vi "Config Read Part Type.vi"(8 "Error In":errorcluster) -> (0 "Error Out":errorcluster, 1 "Part Infos":T1[](array[typedef]), 3 "Part Types":string[](array[string]))   [LabVIEW 2018]
uses:
  type defs/EOL Part Setup.ctl
  02.Type Def's/All Communication Types.ctl
  type defs/Communication with Motors.ctl
  type defs/RAP Signal Control.ctl
  type defs/EOL Motor Type.ctl
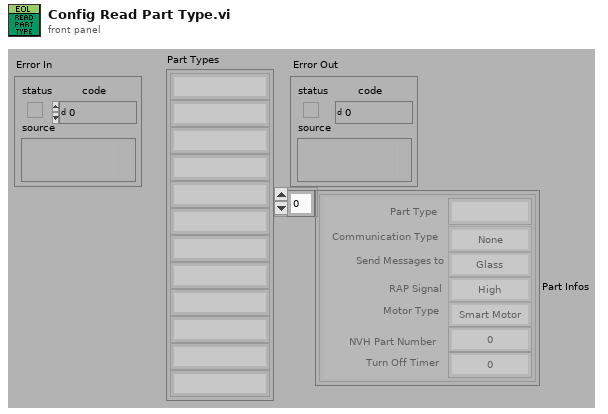
[diagram p1: front panel]
types:
  T1 = typedef "EOL Part Setup.ctl" = cluster{"Communication Type":T2, "Send Messages to":T3, "RAP Signal":T4, "Motor Type":T5, "NVH Part Number":u16, "Turn Off Timer":u16, "Part Type":string}
  T2 = typedef "All Communication Types.ctl" = enum16{"None", "CAN", "RS 232", "RS 232 LIN", "GM LIN", "SnT LIN", "K Line", "Robel CAN", "P42M-Continental", "Inalfa SCU LIN", "Spare 3"}
  T3 = typedef "Communication with Motors.ctl" = enum16{"Glass", "Rollo", "Both"}
  T4 = typedef "RAP Signal Control.ctl" = enum16{"High", "Low", "None"}
  T5 = typedef "EOL Motor Type.ctl" = enum16{"Smart Motor", "Sensor Motor"}
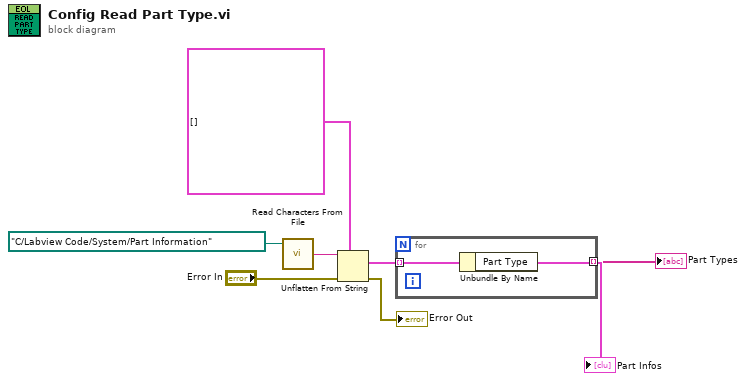
[diagram p0: block diagram]
diagram:
  n1 = call <vilib>:"Read Characters From File.vi"("file path (dialog if empty)"=path "C:/Labview Code/System/Part Information" ("configuration file path")) -> ("character string"=w7:string)  [unwired: 5 in, 3 out]
  n2 = Unflatten From String(type=T1[] [] ("Array"), binary string=w7, error in (no error)="Error In") -> (value=w3:T1[], error out=→"Error Out":errorcluster)  [unwired: 2 in, 1 out]
  "Part Infos" <- w3
  n3 = for {
    tunnel: w3 -> [w9] mode=indexing
    tunnel: [w8] -> w2 mode=indexing
    n4 = Unbundle By Name(w9) -> ("Part Type"=w8:string)
  }
  "Part Types" <- w2
